vi "Protocol Write.vi"(8 "error in (no error)":errorcluster, 10 "data":u8[](array[numeric]), 11 "protocol layer in":refnum<class "TCP.lvclass">) -> (0 "error out":errorcluster, 1 "timed out?":bool, 3 "protocol layer out":refnum<class "TCP.lvclass">)   [LabVIEW 2021, in "TCP.lvclass"]
doc: "Writes to the established TCP connection stored in the class."
uses:
  TCP.lvclass
  TCP.lvclass/TCP.ctl
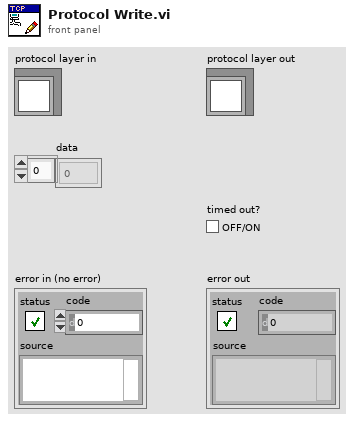
[diagram p1: front panel]
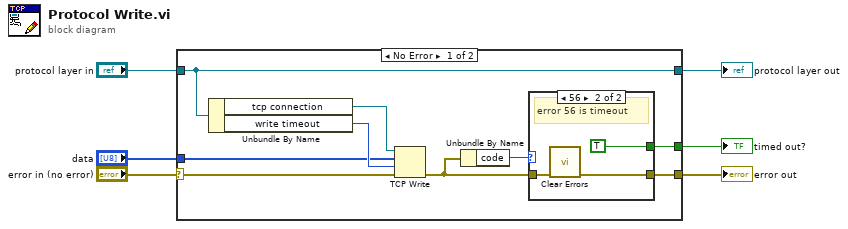
[diagram p0: block diagram]
diagram:
  n1 = case shown="No Error" "error in (no error)" {
    selector: "error in (no error)" -> [w13 w21]
    tunnel: [w15 w21] -> w4
    tunnel: "data" -> [w7 _]
    tunnel: [w11 _] -> w3
    tunnel: "protocol layer in" -> [w9 w20]
    tunnel: [w9 w20] -> w1
    frame No Error {
      n2 = Unbundle By Name(w9) -> ("tcp connection"=w10:refnum<k5>, "write timeout"=w8:i32)
      n3 = TCP Write(connection ID=w10, data in=w7, error in (no error)=w13, 9:w8) -> (error out=w14:errorcluster)  [unwired: 2 out]
      n4 = Unbundle By Name(w14) -> ("code"=w12:i32)
      n5 = case shown="56" w12 {
        tunnel: w14 -> [w16 w18]
        tunnel: [w16 w17] -> w15
        tunnel: [_ TRUE] -> w11
        frame 0, Default {
        }
        frame 56 {
          # "error 56 is timeout"
          n6 = call <vilib>:"Clear Errors.vi"("error in (no error)"=w18) -> ("error out"=w17:errorcluster)  [unwired: 5 in, 1 out]
        }
      }
    }
    frame Error {
    }
  }
  "error out" <- w4
  "protocol layer out" <- w1
  "timed out?" <- w3
